vi "ILMMonitor.vi"() -> ()   [LabVIEW 2016]
uses:
  Equipment/Oxford Software/Oxsoft/BUSGEN.LLB/OxfordAddress.ctl
  Instrument_Setup.vi
  Global/Global Variables/Data_Display_global.vi
panel:
  out "Nitrogen Level":dbl format="%#4_5f"
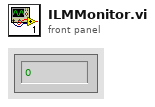
[diagram p1: front panel]
types:
  T1 = typedef "OxfordAddress.ctl" = cluster{"Com Port":i32, "ISOBUS Address":i32, "GPIB Address":i16, "Communication":enum16{"RS232", "ISOBUS", "GPIB", "Gateway"}}
  T2 = typedef "ILMSetup.ctl" = cluster{"Address":T1, "ILM Name":string, "Display Channel":i32[]}
  T3 = typedef "LambdaSetup.ctl" = cluster{"Address":T1, "Max 4.2K temp":dbl[unit], "Max 2.2K temp":dbl[unit]}
  T4 = typedef "ILMChannelStatus.ctl" = cluster{"Probe current":bool, "Probe fast":bool, "Probe slow":bool, "Auto-fill":enum16{"End fill", "Not filling", "Filling", "Start filling"}, "Fill":bool, "Low level":bool, "Alm requested":bool, "Pre-pulse I":bool}
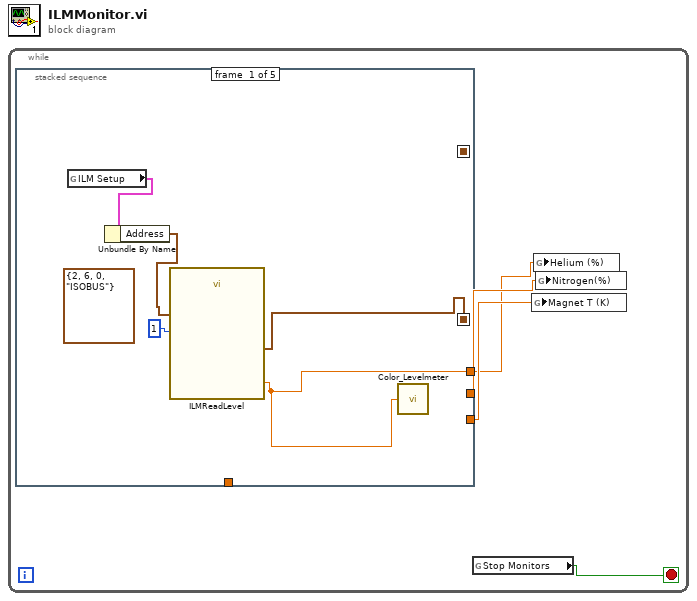
[diagram p0: block diagram]
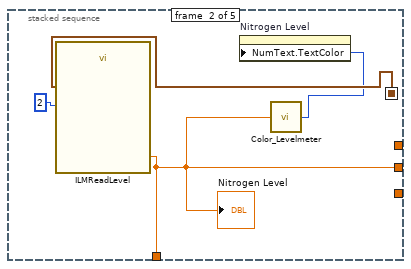
[diagram p2: hidden frame]
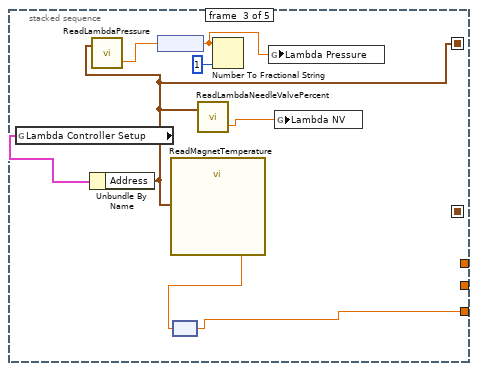
[diagram p3: hidden frame]
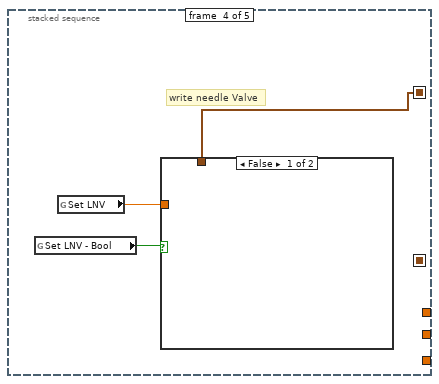
[diagram p4: hidden frame]
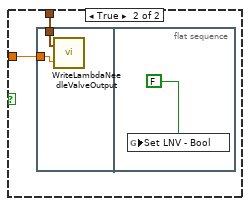
[diagram p5: hidden frame]
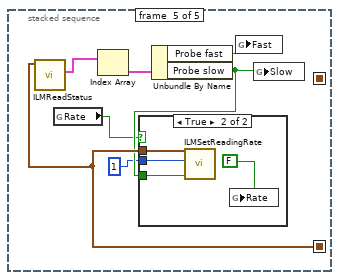
[diagram p6: hidden frame]
diagram:
  n1 = while {
    stop <- w4 stop-if-true
    n2 = stacked-sequence {
      seq-local: [w8 _ _ _ _] -> [_ w12 _ _ w36]
      seq-local: [_ _ w14 _ _] -> [_ _ _ w24 _]
      tunnel: [_ w10 _ _ _] -> _
      tunnel: [_ _ w20 _ _] -> w3
      tunnel: [_ w10 _ _ _] -> w2
      tunnel: [w7 _ _ _ _] -> w1
      frame #0 {
        (unwired) T1 {"Com Port"=2, "ISOBUS Address"=6, "GPIB Address"=0, "Communication"=enum."ISOBUS"} ("Address")
        n3 = global read "Instrument_Setup.vi" "ILM Setup"() -> (w6:T2)
        n4 = Unbundle By Name(w6) -> ("Address"=w5:T1)
        n5 = call "ILMReadLevel.vi"("Address"=w5, "Channel number (1-3)"=u8 1) -> ("Address(thru)"=w8:T1, "Level"=w7:dbl)  [unwired: 1 out]
        n6 = call "Color_Levelmeter.vi"("In"=w7) -> ()  [unwired: 1 out]
      }
      frame #1 {
        n7 = call "ILMReadLevel.vi"("Address"=w12, "Channel number (1-3)"=u8 2) -> ("Level"=w10:dbl)  [unwired: 2 out]
        "Nitrogen Level" <- w10
        n8 = call "Color_Levelmeter.vi"("In"=w10) -> ("Out"=w11:i32)
        n9 = property on="Nitrogen Level" class="DigNum (strict)"("NumText.TextColor"=w11) -> ()  [unwired: 2 in, 2 out]
      }
      frame #2 {
        n10 = global read "Instrument_Setup.vi" "Lambda Controller Setup"() -> (w15:T3)
        n11 = Unbundle By Name(w15) -> ("Address"=w14:T1)
        n12 = call "ReadLambdaPressure.vi"("Address"=w14) -> ("Pressure"=w18:dbl[unit])  [unwired: 1 in, 1 out]
        n13 = node(w18) -> (w16:dbl)
        n14 = call "ReadMagnetTemperature.vi"("Address"=w14) -> ("Magnet Temperature"=w21:dbl[unit])  [unwired: 1 in, 1 out]
        n15 = node(w21) -> (w20:dbl)
        n16 = call "ReadLambdaNeedleValvePercent.vi"("Address"=w14) -> ("Actual Needle Valve  %"=w17:dbl)  [unwired: 1 in, 1 out]
        n17 = Number To Fractional String(number=w16, precision (6)=1) -> ()  [unwired: 2 in, 1 out]
        n18 = global write "Data_Display_global.vi" "Lambda Pressure"(w16) -> ()
        n19 = global write "Data_Display_global.vi" "Lambda NV"(w17) -> ()
      }
      frame #3 {
        # "write needle Valve"
        n20 = global read "Data_Display_global.vi" "Set LNV - Bool"() -> (w22:bool)
        n21 = global read "Data_Display_global.vi" "Set LNV"() -> (w23:dbl)
        n22 = case shown="False" w22 {
          tunnel: w24 -> [_ w26]
          tunnel: w23 -> [_ w25]
          frame False {
          }
          frame True {
            n23 = flat-sequence {
              tunnel: w26 -> [w28]
              tunnel: w25 -> [w27]
              frame #0 {
                n24 = call "WriteLambdaNeedleValveOutput.vi"("Needle Valve Output (%)"=w27, "Address"=w28) -> ()  [unwired: 1 in, 1 out]
              }
              frame #1 {
                n25 = global write "Data_Display_global.vi" "Set LNV - Bool"(FALSE) -> ()
              }
            }
          }
        }
      }
      frame #4 {
        n26 = call "ILMReadStatus.vi"("Instrument address"=w36) -> ("Channel"=w35:T4[])  [unwired: 3 in, 3 out]
        n27 = global read "Data_Display_global.vi" "Rate"() -> (w30:bool)
        n28 = Index Array(array=w35) -> (element=w34:T4)  [unwired: 1 in]
        n29 = Unbundle By Name(w34) -> ("Probe fast"=w33:bool, "Probe slow"=w32:bool)
        n30 = case shown="True" w30 {
          tunnel: w32 -> [_ w40]
          tunnel: w36 -> [_ w39]
          tunnel: 1 -> [_ w38]
          frame False {
          }
          frame True {
            n31 = call "ILMSetReadingRate.vi"("Fast"=w40, "Channel(1-3)"=w38, "Address"=w39) -> ()  [unwired: 1 out]
            n32 = global write "Data_Display_global.vi" "Rate"(FALSE) -> ()
          }
        }
        n33 = global write "Data_Display_global.vi" "Fast"(w33) -> ()
        n34 = global write "Data_Display_global.vi" "Slow"(w32) -> ()
      }
    }
    n35 = global read "Data_Display_global.vi" "Stop Monitors"() -> (w4:bool)
    n36 = global write "Data_Display_global.vi" "Magnet T (K)"(w3) -> ()
    n37 = global write "Data_Display_global.vi" "Helium (%)"(w1) -> ()
    n38 = global write "Data_Display_global.vi" "Nitrogen(%)"(w2) -> ()
  }
